vi "rea_Mazak_create_output.vi"(9 "error in":errorcluster, 10 "URL":string, 11 "Folder Name":path=path "C:/Users/me1ssv/Music/MTConnect") -> (0 "error out":errorcluster, 1 "Triggger G1,G2, or G3":bool, 2 "output cluster":T1, 3 "Array":dbl[][](array[numeric]), 4 "NC code":string="\n", 5 "SLoad":dbl, 7 "Feed":dbl)   [LabVIEW 2014]
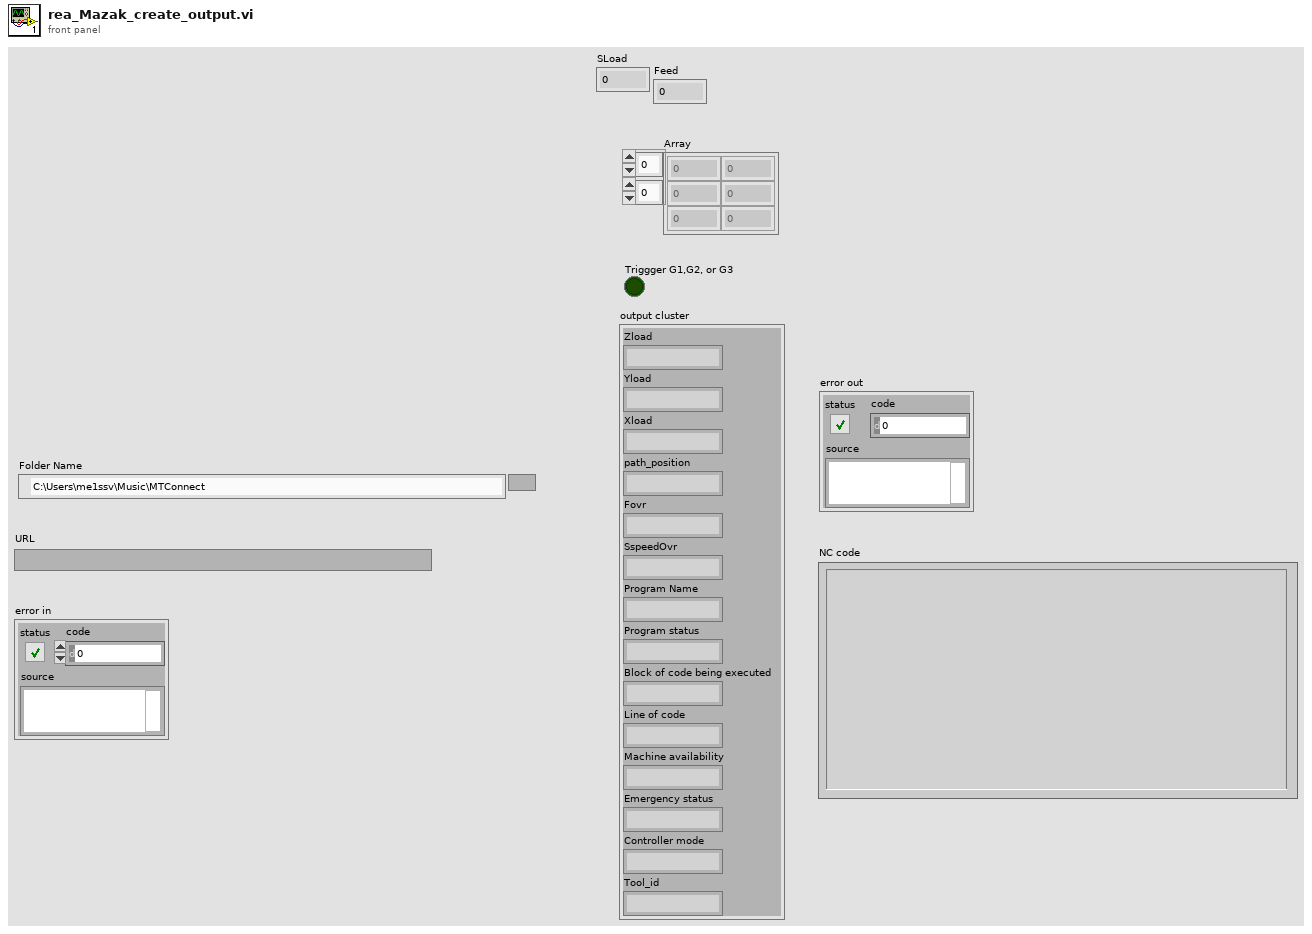
[diagram p1: front panel]
types:
  T1 = cluster{"Zload":string, "Yload":string, "Xload":string, "path_position":string, "Fovr":string, "SspeedOvr":string, "Program Name":string, "Program status":string, "Block of code being executed":string, "Line of code":string, "Machine availability":string, "Emergency status":string, "Controller mode":string, "Tool_id":string}
  T2 = cluster{"EmergencyStop":string, "Availability":string, "PowerState":string, "Fact":string, "Fovr":string, "Frapidovr":string, "Execution":string, "Line":string, "ControllerMode":string, "PartCount":string, "Program":string, "ToolNumber":string}
  T3 = cluster{"c_AngularVelocity":string, "c_Load_Cload":string, "c_Angle":string, "c_RotaryMode":string, "c_Temperature":string, "c_Load_Sload":string, "c_RotaryVelocity_Srpm":string, "c_RotaryVelocity_Sovr":string}
  T4 = cluster{"xPosition":string, "xLoad":string, "yPosition":string, "yLoad":string, "zPosition":string, "zLoad":string}
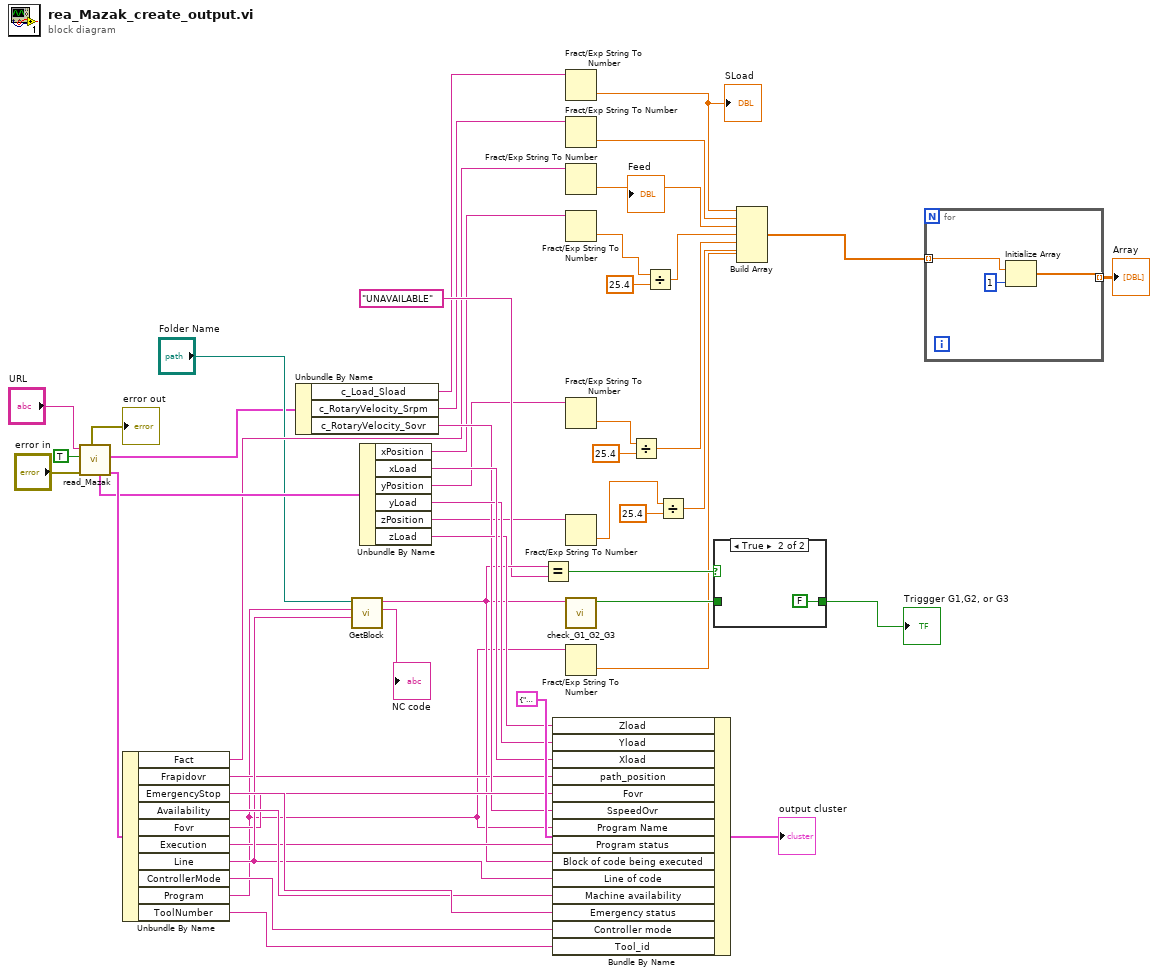
[diagram p0: block diagram]
diagram:
  n1 = call "read_Mazak.vi"("error in"="error in", "Boolean"=TRUE, "URL"="URL") -> ("machine"=w48:T2, "c"=w13:T3, "position"=w40:T4, "error out"=→"error out":errorcluster)  [unwired: 2 in, 3 out]
  n2 = Unbundle By Name(w48) -> ("Fact"=w24:string, "Frapidovr"=w35:string, "EmergencyStop"=w47:string, "Availability"=w46:string, "Fovr"=w41:string, "Execution"=w42:string, "Line"=w45:string, "ControllerMode"=w44:string, "Program"=w11:string, "ToolNumber"=w43:string)
  n3 = Unbundle By Name(w13) -> ("c_Load_Sload"=w27:string, "c_RotaryVelocity_Srpm"=w26:string, "c_RotaryVelocity_Sovr"=w36:string)
  n4 = call "GetBlock.vi"("Line"=w45, "Program Number"=w11, "Folder Name"="Folder Name") -> ("Tool Data"=→"NC code":string, "Block"=w34:string)  [unwired: 7 in]
  n5 = Unbundle By Name(w40) -> ("xPosition"=w29:string, "xLoad"=w39:string, "yPosition"=w28:string, "yLoad"=w38:string, "zPosition"=w12:string, "zLoad"=w37:string)
  n6 = Equal?(x=w34, y="UNAVAILABLE") -> (x = y?=w32:bool)
  n7 = Bundle By Name(cluster=T1 {"Zload"="", "Yload"="", "Xload"="", "path_position"="", "Fovr"="", "SspeedOvr"="", "Program Name"="", "Program status"="", "Block of code being executed"="", "Line of code"="", "Machine availability"="", "Emergency status"="", "Controller mode"="", "Tool_id"=""} ("Machine Data"), "Zload"=w37, "Yload"=w38, "Xload"=w39, "path_position"=w35, "Fovr"=w41, "SspeedOvr"=w36, "Program Name"=w11, "Program status"=w42, "Block of code being executed"=w34, "Line of code"=w45, "Machine availability"=w46, "Emergency status"=w47, "Controller mode"=w44, "Tool_id"=w43) -> (→"output cluster":T1)
  n8 = Fract/Exp String To Number(string=w27) -> (number=w14:dbl)  [unwired: 3 in, 1 out]
  "SLoad" <- w14
  n9 = Fract/Exp String To Number(string=w26) -> (number=w25:dbl)  [unwired: 3 in, 1 out]
  n10 = Fract/Exp String To Number(string=w24) -> (number=w23:dbl)  [unwired: 3 in, 1 out]
  "Feed" <- w23
  n11 = Fract/Exp String To Number(string=w29) -> (number=w7:dbl)  [unwired: 3 in, 1 out]
  n12 = Fract/Exp String To Number(string=w28) -> (number=w5:dbl)  [unwired: 3 in, 1 out]
  n13 = Fract/Exp String To Number(string=w12) -> (number=w2:dbl)  [unwired: 3 in, 1 out]
  n14 = call "check_G1_G2_G3.vi"("current line"=w34) -> ("Triggger G1,G2, or G3"=w31:bool)  [unwired: 8 in, 1 out]
  n15 = Fract/Exp String To Number(string=w11) -> (number=w22:dbl)  [unwired: 3 in, 1 out]
  n16 = Divide(x=w5, y=25.4) -> (x/y=w4:dbl)
  n17 = Divide(x=w7, y=25.4) -> (x/y=w8:dbl)
  n18 = Divide(x=w2, y=25.4) -> (x/y=w1:dbl)
  n19 = case shown="True" w32 {
    tunnel: [w51 FALSE ("Triggger G1,G2, or G3")] -> w30
    tunnel: w31 -> [w51 _]
    frame False {
    }
    frame True {
    }
  }
  "Triggger G1,G2, or G3" <- w30
  n20 = Build Array(w14, w25, w23, w8, w4, w1, w22) -> (w18:dbl[])
  n21 = for {
    tunnel: w18 -> [w54] mode=indexing
    tunnel: [w53] -> w17 mode=indexing
    n22 = Initialize Array(w54, 1 ("dimension size")) -> (w53:dbl[])
  }
  "Array" <- w17
